vi "CustomerSpecific_SendReceive.vi"(6 "error source":string="Diagnostic Service.vi", 8 "error in (no error)":errorcluster, 9 "data in":u8[](array[numeric]), 10 "require response?":bool=TRUE, 11 "diag ref in":T1={"Diag CAN Handle"=0, "Transport Protocol"=enum."ISO TP - Normal Mode", "Receive Address Extension"=0, "Transmit Address Extension"=0, "Receive CAN Id"=0, "Transmit CAN Id"=0, "Log Frames ?"=FALSE, "My TP Address"=0, "Other TP Address"=0, "T1"=0, "T2"=0, "T3"=0, "T4"=0, "Tx SN"=0, "Block Size"=0, "Rx SN"=0, "VW TP Initialized?"=FALSE, "Tx block no"=0, "baud rate"=0, "Interface"="", "Channel Diag CAN Handle"=0, "UDP Connection ID"=refnum, "TCP Connection ID"=refnum, "Target IP Addr"=0, "Source Address"=0, "Target Address"=0, "Send Header NACK?"=FALSE, "DLL Handle"=0, "NAD"=0, "Time Stamp read first"=0.0, "Time Stamp read last"=0.0, "Time Stamp write first"=0.0, "Time Stamp write last"=0.0, "Time Stamp write"=0.0, "Time Stamp read"=0.0, " I/O Mode"=0, "FD Baudrate"=0, "TX_DL"=8, "RX_DL"=8, "DoIP Protocol Version"=1, " Selected I/O Mode"=0, "TesterPresent Counter"=0, "TesterPresent Limit"=0, "TesterPresent Tick[ms]"=10, "TesterPresent RequireResponse?"=FALSE, "TesterPresent Stored Ref?"=FALSE, "TesterPresent Message"=[], "TesterPresent Task Handle"=0, "TesterPresent Semaphore"=refnum, "Response Plausibility Check"=1, "Default Version?"=TRUE, "Diagostic Globals"={"Timeout FC (Bs)"=250, "Timeout CF (Cr)"=250, "Timeout Diag Command"=1000, "Receive Block Size (BS)"=0, "Wait Time CF (STmin)"=5, "Max Waits (N_WFTmax)"=10, "Waits to Send (N_WAIT)"=0, "Time between Waits (TW)"=25, "Fill CAN Frames?"=TRUE, "Fill Byte"=255, "Invalid Response as Error?"=FALSE, "Max RspPending Count"=5, "VWTP Command Timeout"=50, "Transport Protocol"=enum."Diagnostics on IP", "Diag CAN Handle"=0, "DLL Handle"=0, "Timeout RspPending"=1000}, "Session-based Properties?"=FALSE, "NI-XNET IP Stack Reference"=0, "NI-XNET IP Stack TCP Reference"=-1, "NI-XNET IP Stack UDP Reference"=-1, "NI-XNET IP Stack Local Interface"="", "Functional CAN Id"=0, "Diag CAN Queue"=refnum, "Frame Fillling Mode"=0, "DoIP Acknowledge Mode"=0, "Message Buffer"=[]} {"Diagostic Globals"."Fill Byte" format="%x"; "TesterPresent Message" format="%.0x"; "Selected I/O Mode" items=["CAN", "CAN FD", "CAN FD+BRS", "ECU Determined"]; "DoIP Protocol Version" items=["2010"=1, "2012"=2]; "RX_DL" items=["8"=8, "12"=12, "16"=16, "20"=20, "24"=24, "32"=32, "48"=48, "64"=64]; "TX_DL" items=["8"=8, "12"=12, "16"=16, "20"=20, "24"=24, "32"=32, "48"=48, "64"=64]; "I/O Mode" items=["CAN", "CAN FD", "CAN FD+BRS", "Not yet determined"]}) -> (0 "error out":errorcluster, 1 "data out":u8[](array[numeric]), 2 "error code":u8, 3 "diag ref out":T1={"Diag CAN Handle"=0, "Transport Protocol"=enum."ISO TP - Normal Mode", "Receive Address Extension"=0, "Transmit Address Extension"=0, "Receive CAN Id"=0, "Transmit CAN Id"=0, "Log Frames ?"=FALSE, "My TP Address"=0, "Other TP Address"=0, "T1"=0, "T2"=0, "T3"=0, "T4"=0, "Tx SN"=0, "Block Size"=0, "Rx SN"=0, "VW TP Initialized?"=FALSE, "Tx block no"=0, "baud rate"=0, "Interface"="", "Channel Diag CAN Handle"=0, "UDP Connection ID"=refnum, "TCP Connection ID"=refnum, "Target IP Addr"=0, "Source Address"=0, "Target Address"=0, "Send Header NACK?"=FALSE, "DLL Handle"=0, "NAD"=0, "Time Stamp read first"=0.0, "Time Stamp read last"=0.0, "Time Stamp write first"=0.0, "Time Stamp write last"=0.0, "Time Stamp write"=0.0, "Time Stamp read"=0.0, " I/O Mode"=0, "FD Baudrate"=0, "TX_DL"=8, "RX_DL"=8, "DoIP Protocol Version"=1, " Selected I/O Mode"=0, "TesterPresent Counter"=0, "TesterPresent Limit"=0, "TesterPresent Tick[ms]"=10, "TesterPresent RequireResponse?"=FALSE, "TesterPresent Stored Ref?"=FALSE, "TesterPresent Message"=[], "TesterPresent Task Handle"=0, "TesterPresent Semaphore"=refnum, "Response Plausibility Check"=1, "Default Version?"=TRUE, "Diagostic Globals"={"Timeout FC (Bs)"=250, "Timeout CF (Cr)"=250, "Timeout Diag Command"=1000, "Receive Block Size (BS)"=0, "Wait Time CF (STmin)"=5, "Max Waits (N_WFTmax)"=10, "Waits to Send (N_WAIT)"=0, "Time between Waits (TW)"=25, "Fill CAN Frames?"=TRUE, "Fill Byte"=255, "Invalid Response as Error?"=FALSE, "Max RspPending Count"=5, "VWTP Command Timeout"=50, "Transport Protocol"=enum."Diagnostics on IP", "Diag CAN Handle"=0, "DLL Handle"=0, "Timeout RspPending"=1000}, "Session-based Properties?"=FALSE, "NI-XNET IP Stack Reference"=0, "NI-XNET IP Stack TCP Reference"=-1, "NI-XNET IP Stack UDP Reference"=-1, "NI-XNET IP Stack Local Interface"="", "Functional CAN Id"=0, "Diag CAN Queue"=refnum, "Frame Fillling Mode"=0, "DoIP Acknowledge Mode"=0, "Message Buffer"=[]} {"Diagostic Globals"."Fill Byte" format="%x"; "TesterPresent Message" format="%.0x"; "Selected I/O Mode" items=["CAN", "CAN FD", "CAN FD+BRS", "ECU Determined"]; "DoIP Protocol Version" items=["2010"=1, "2012"=2]; "RX_DL" items=["8"=8, "12"=12, "16"=16, "20"=20, "24"=24, "32"=32, "48"=48, "64"=64]; "TX_DL" items=["8"=8, "12"=12, "16"=16, "20"=20, "24"=24, "32"=32, "48"=48, "64"=64]; "I/O Mode" items=["CAN", "CAN FD", "CAN FD+BRS", "Not yet determined"]})   [LabVIEW 2024, in "Diagnostics Addon Engine.lvlib"]
uses:
  Diagnostics Addon Engine.lvlib
  <vilib>/Automotive Diagnostic Command Set/Diagnostic Transport.llb/Diag Reference.ctl
  <vilib>/Automotive Diagnostic Command Set/Diagnostic Transport.llb/Transport Protocol Selector.ctl
  <vilib>/Automotive Diagnostic Command Set/Diagnostic Transport.llb/DoIP Protocol Version.ctl
  <vilib>/Automotive Diagnostic Command Set/Diagnostic Transport.llb/Diag Globals.ctl
  <vilib>/Automotive Diagnostic Command Set/Diagnostic Transport.llb/ISOTP Recv Frame.vi
  <vilib>/Automotive Diagnostic Command Set/Diagnostic Transport.llb/ISOTP Recv CFs.vi
  <vilib>/Automotive Diagnostic Command Set/Diagnostic Transport.llb/ISOTP7 Recv Frame.vi
  <vilib>/Automotive Diagnostic Command Set/Diagnostic Transport.llb/ISOTP7 Recv CFs.vi
  <vilib>/Automotive Diagnostic Command Set/Diagnostic Transport.llb/ISOTP Send FF.vi
  <vilib>/Automotive Diagnostic Command Set/Diagnostic Transport.llb/ISOTP Send CFs.vi
  <vilib>/Automotive Diagnostic Command Set/Diagnostic Transport.llb/ISOTP Send Single Frame.vi
  <vilib>/Automotive Diagnostic Command Set/Diagnostic Transport.llb/Long CAN Frame Forced.vi
  <vilib>/Automotive Diagnostic Command Set/Diagnostic Transport.llb/ISOTP7 Send FF.vi
  <vilib>/Automotive Diagnostic Command Set/Diagnostic Transport.llb/ISOTP7 Send CFs.vi
  <vilib>/Automotive Diagnostic Command Set/Diagnostic Transport.llb/ISOTP7 Send Single Frame.vi
  <vilib>/Automotive Diagnostic Command Set/Diagnostic Transport.llb/ISOTP Check Redo.vi
  <vilib>/Automotive Diagnostic Command Set/Diagnostic Transport.llb/ISOTP Recv Block.vi
  <vilib>/Automotive Diagnostic Command Set/Diagnostic Transport.llb/ISOTP7 Recv Block.vi
  <vilib>/Automotive Diagnostic Command Set/Diagnostic Transport.llb/ISOTP Send Frame.vi
  <vilib>/Automotive Diagnostic Command Set/Diagnostic Transport.llb/ISOTP Recv FC.vi
  <vilib>/Automotive Diagnostic Command Set/Diagnostic Transport.llb/ISOTP Send CF.vi
  <vilib>/Automotive Diagnostic Command Set/Diagnostic Transport.llb/Diag Fill Frame.vi
  <vilib>/Automotive Diagnostic Command Set/Diagnostic Transport.llb/ISOTP Calc Send Params.vi
  <vilib>/Automotive Diagnostic Command Set/Diagnostic Transport.llb/Diag Get Globals.vi
  <vilib>/Automotive Diagnostic Command Set/Diagnostic Transport.llb/ISOTP7 Send Frame.vi
  <vilib>/Automotive Diagnostic Command Set/Diagnostic Transport.llb/ISOTP7 Recv FC.vi
  <vilib>/Automotive Diagnostic Command Set/Diagnostic Transport.llb/ISOTP7 Send CF.vi
  <vilib>/Automotive Diagnostic Command Set/Diagnostic Transport.llb/ISOTP Send FC.vi
  <vilib>/Automotive Diagnostic Command Set/Diagnostic Transport.llb/ISOTP Add CF.vi
  <vilib>/Automotive Diagnostic Command Set/Diagnostic Transport.llb/ISOTP7 Send FC.vi
  <vilib>/Automotive Diagnostic Command Set/Diagnostic Transport.llb/ISOTP7 Add CF.vi
  <vilib>/Automotive Diagnostic Command Set/Diagnostic Transport.llb/Diag Globals.vi
  <vilib>/Automotive Diagnostic Command Set/Diagnostic Transport.llb/CAN Send Frame Check Queue.vi
  <vilib>/Automotive Diagnostic Command Set/Diagnostic Transport.llb/Diag CAN get timestamp.vi
  <vilib>/Automotive Diagnostic Command Set/Diagnostic Transport.llb/Diag CAN read.vi
  <vilib>/Automotive Diagnostic Command Set/Diagnostic Transport.llb/ISOTP Calc Actual IO Mode.vi
  <vilib>/Automotive Diagnostic Command Set/Diagnostic Transport.llb/ISOTP Get FC Data.vi
  <vilib>/addons/Automotive Diagnostic Command Set/NI_Automotive Diagnostic Command Set.lvlib
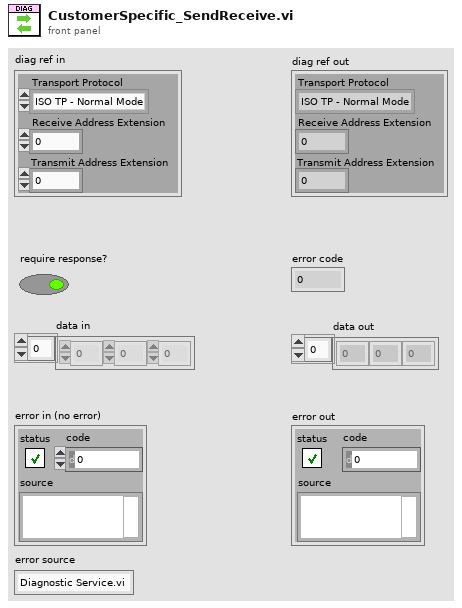
[diagram p1: front panel]
types:
  T1 = typedef "NI_Automotive Diagnostic Command Set.lvlib/Diag Reference.ctl" = cluster{"Diag CAN Handle":u32, "Transport Protocol":T2, "Receive Address Extension":u8, "Transmit Address Extension":u8, "Receive CAN Id":u32, "Transmit CAN Id":u32, "Log Frames ?":bool, "My TP Address":u8, "Other TP Address":u8, "T1":u16, "T2":u16, "T3":u16, "T4":u16, "Tx SN":u8, "Block Size":u8, "Rx SN":u8, "VW TP Initialized?":bool, "Tx block no":u8, "baud rate":u64, "Interface":string, "Channel Diag CAN Handle":u32, "UDP Connection ID":refnum<k16>, "TCP Connection ID":refnum<k5>, "Target IP Addr":u32, "Source Address":u16, "Target Address":u16, "Send Header NACK?":bool, "DLL Handle":u32, "NAD":u8, "Time Stamp read first":dbl, "Time Stamp read last":dbl, "Time Stamp write first":dbl, "Time Stamp write last":dbl, "Time Stamp write":dbl, "Time Stamp read":dbl, " I/O Mode":u32, "FD Baudrate":u64, "TX_DL":u16, "RX_DL":u16, "DoIP Protocol Version":T3, " Selected I/O Mode":u32, "TesterPresent Counter":u32, "TesterPresent Limit":u32, "TesterPresent Tick[ms]":i32, "TesterPresent RequireResponse?":bool, "TesterPresent Stored Ref?":bool, "TesterPresent Message":u8[], "TesterPresent Task Handle":i32, "TesterPresent Semaphore":T4, "Response Plausibility Check":u32, "Default Version?":bool, "Diagostic Globals":T5, "Session-based Properties?":bool, "NI-XNET IP Stack Reference":i64, "NI-XNET IP Stack TCP Reference":i64, "NI-XNET IP Stack UDP Reference":i64, "NI-XNET IP Stack Local Interface":string, "Functional CAN Id":u32, "Diag CAN Queue":refnum<queue>, "Frame Fillling Mode":u32, "DoIP Acknowledge Mode":u32, "Message Buffer":u8[]}
  T2 = typedef "NI_Automotive Diagnostic Command Set.lvlib/Transport Protocol Selector.ctl" = enum16{"ISO TP - Normal Mode", "ISO TP - Mixed Mode", "VW TP 2.0", "Diagnostics on IP", "ISO TP LIN"}
  T3 = typedef "NI_Automotive Diagnostic Command Set.lvlib/DoIP Protocol Version.ctl" = u8
  T4 = typedef "Semaphore RefNum" = refnum<k1>
  T5 = typedef "NI_Automotive Diagnostic Command Set.lvlib/Diag Globals.ctl" = cluster{"Timeout FC (Bs)":u32, "Timeout CF (Cr)":u32, "Timeout Diag Command":u32, "Receive Block Size (BS)":u8, "Wait Time CF (STmin)":u8, "Max Waits (N_WFTmax)":u8, "Waits to Send (N_WAIT)":i32, "Time between Waits (TW)":u32, "Fill CAN Frames?":bool, "Fill Byte":u32, "Invalid Response as Error?":bool, "Max RspPending Count":u32, "VWTP Command Timeout":u32, "Transport Protocol":T2, "Diag CAN Handle":u32, "DLL Handle":u32, "Timeout RspPending":u32}
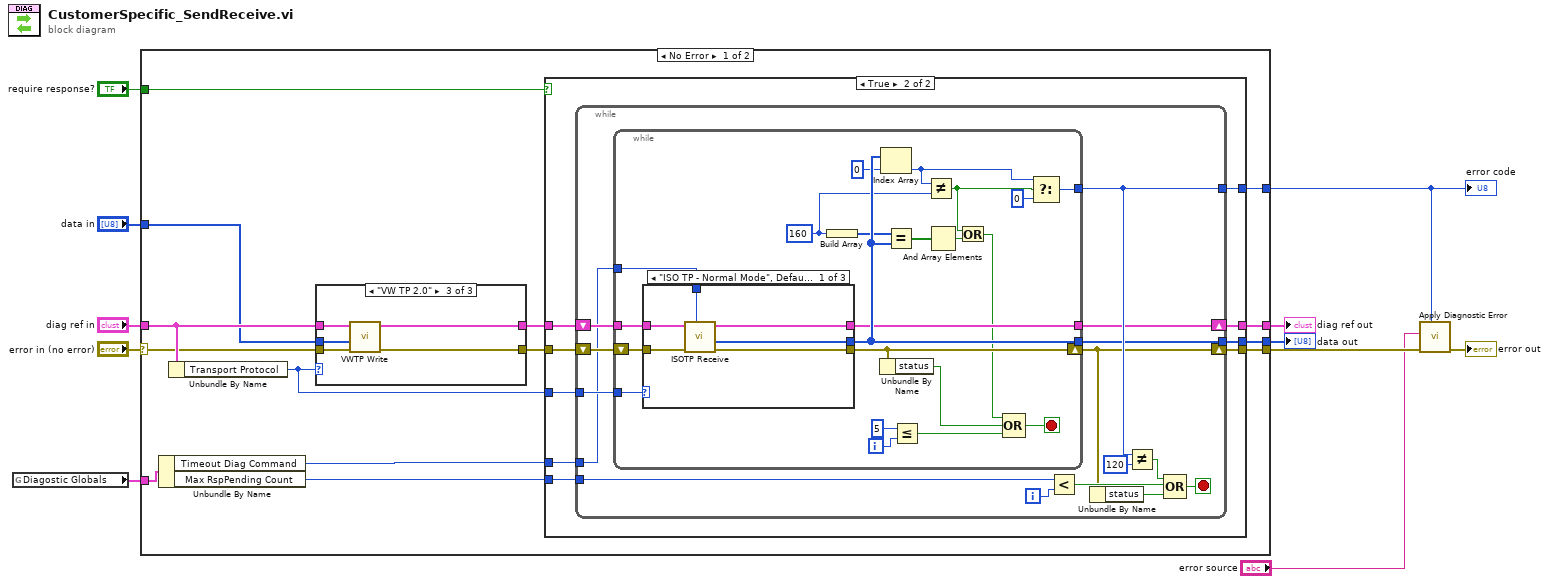
[diagram p0: block diagram]
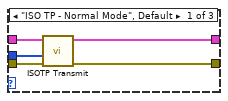
[diagram p2: hidden frame]
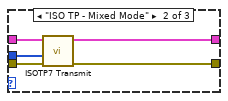
[diagram p3: hidden frame]
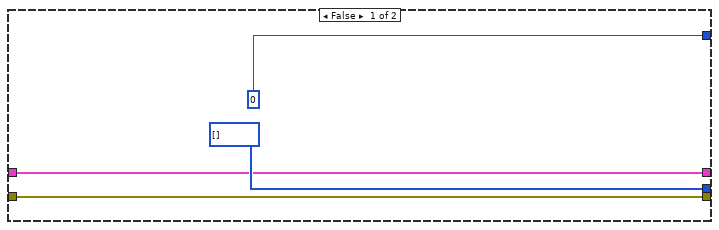
[diagram p4: hidden frame]
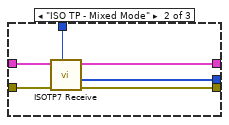
[diagram p5: hidden frame]
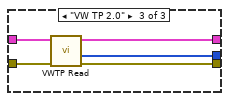
[diagram p6: hidden frame]
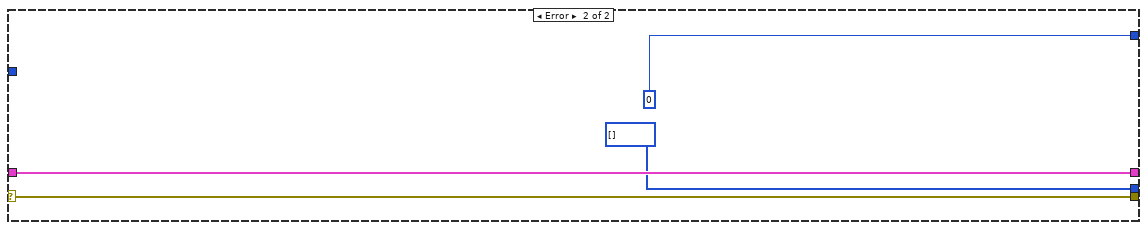
[diagram p7: hidden frame]
diagram:
  n1 = global read "Diag Globals.vi" "Diagostic Globals"() -> (w2:T5)
  n2 = case shown="No Error" "error in (no error)" {
    selector: "error in (no error)" -> [w19 w110]
    tunnel: "data in" -> [w18 _]
    tunnel: [w25 u8[] [] ("data out")] -> w5
    tunnel: [w24 w111] -> w1
    tunnel: [w23 w110] -> w11
    tunnel: "diag ref in" -> [w20 w111]
    tunnel: [w22 u8 0 ("error code")] -> w8
    tunnel: "require response?" -> [w21 _]
    tunnel: w2 -> [w15 _]
    frame No Error {
      n3 = Unbundle By Name(w15) -> ("Timeout Diag Command"=w12:u32, "Max RspPending Count"=w14:u32)
      n4 = Unbundle By Name(w20) -> ("Transport Protocol"=w13:T2)
      n5 = case shown="\"VW TP 2.0\"" w13 {
        tunnel: w19 -> [w30 w35 w39]
        tunnel: w18 -> [w29 w34 w36]
        tunnel: [w27 w32 w38] -> w16
        tunnel: w20 -> [w28 w33 w40]
        tunnel: [w26 w31 w37] -> w17
        frame "ISO TP - Normal Mode", Default {
          n6 = call <vilib>:"ISOTP Transmit.vi"("error in (no error)"=w30, "data"=w29, "diag ref in"=w28) -> ("error out"=w26:errorcluster, "diag ref out"=w27:T1)  [unwired: 7 in]
        }
        frame "ISO TP - Mixed Mode" {
          n7 = call <vilib>:"ISOTP7 Transmit.vi"("error in (no error)"=w35, "data"=w34, "diag ref in"=w33) -> ("error out"=w31:errorcluster, "diag ref out"=w32:T1)  [unwired: 7 in]
        }
        frame "VW TP 2.0" {
          n8 = call <vilib>:"VWTP Write.vi"("error in"=w39, "data in"=w36, "diag ref in"=w40) -> ("error out"=w37:errorcluster, "diag ref out"=w38:T1)  [unwired: 7 in]
        }
      }
      n9 = case shown="True" w21 {
        tunnel: [u8[] [] ("data out") w53] -> w25
        tunnel: [w43 w52] -> w24
        tunnel: [w42 w51] -> w23
        tunnel: w16 -> [w43 w50]
        tunnel: w17 -> [w42 w49]
        tunnel: [u8 0 ("error code") w48] -> w22
        tunnel: w14 -> [_ w47]
        tunnel: w13 -> [_ w46]
        tunnel: w12 -> [_ w45]
        frame False {
        }
        frame True {
          n10 = while {
            tunnel: [w58] -> w53
            shift-right: [w57] -> w51
            shift-left: w49 -> [w61]
            tunnel: [w59] -> w48
            shift-right: [w56] -> w52
            shift-left: w50 -> [w60]
            tunnel: w47 -> [w62]
            tunnel: w46 -> [w55]
            tunnel: w45 -> [w54]
            i -> [w64]
            stop <- w67 stop-if-true
            n11 = while {
              tunnel: [w84] -> w58
              tunnel: [w81] -> w56
              tunnel: w60 -> [w85]
              tunnel: [w83] -> w59
              shift-right: [w82] -> w57
              shift-left: w61 -> [w86]
              tunnel: w55 -> [w78]
              tunnel: w54 -> [w77]
              i -> [w87]
              stop <- w90 stop-if-true
              w75 = u8 160 ("element")
              n12 = case shown="\"ISO TP - Normal Mode\", Default" w78 {
                tunnel: w86 -> [w91 w97 w106]
                tunnel: [w96 w102 w103] -> w84
                tunnel: [w95 w101 w104] -> w81
                tunnel: w85 -> [w92 w98 w107]
                tunnel: [w94 w100 w105] -> w82
                tunnel: w77 -> [w93 w99 _]
                frame "ISO TP - Normal Mode", Default {
                  n13 = call <vilib>:"ISOTP Receive.vi"("timeout [ms]"=w93, "error in (no error)"=w91, "diag ref in"=w92) -> ("error out"=w94:errorcluster, "data"=w96:u8[], "diag ref out"=w95:T1)  [unwired: 6 in]
                }
                frame "ISO TP - Mixed Mode" {
                  n14 = call <vilib>:"ISOTP7 Receive.vi"("timeout [ms]"=w99, "error in (no error)"=w97, "diag ref in"=w98) -> ("error out"=w100:errorcluster, "data"=w102:u8[], "diag ref out"=w101:T1)  [unwired: 6 in]
                }
                frame "VW TP 2.0" {
                  n15 = call <vilib>:"VWTP Read.vi"("error in"=w106, "diag ref in"=w107) -> ("error out"=w105:errorcluster, "data out"=w103:u8[], "diag ref out"=w104:T1)  [unwired: 7 in]
                }
              }
              n16 = Build Array(w75) -> (w76:u8[])
              n17 = Unbundle By Name(w82) -> ("status"=w79:bool)
              n18 = Index Array(array=w84, index=0) -> (element=w70:u8)
              n19 = Equal?(x=w76, y=w84) -> (x = y?=w73:bool[])
              n20 = Less Or Equal?(x=5, y=w87) -> (x <= y?=w88:bool)
              n21 = Not Equal?(x=w70, y=w75) -> (x != y?=w71:bool)
              n22 = And Array Elements(Boolean array=w73) -> (logical AND=w72:bool)
              n23 = Or(x=w71, y=w72) -> (x .or. y?=w80:bool)
              n24 = Compound Arithmetic op=OR(w80, w79, w88) -> (w90:bool)
              n25 = Select(t=w70, s=w71, f=u8 0) -> (s? t:f=w83:u8)
            }
            n26 = Less?(x=w62, y=w64) -> (x < y?=w63:bool)
            n27 = Unbundle By Name(w57) -> ("status"=w66:bool)
            n28 = Not Equal?(x=w59, y=u8 120) -> (x != y?=w65:bool)
            n29 = Compound Arithmetic op=OR(w65, w63, w66) -> (w67:bool)
          }
        }
      }
    }
    frame Error {
    }
  }
  "data out" <- w5
  "error code" <- w8
  "diag ref out" <- w1
  n30 = call <vilib>:"Apply Diagnostic Error.vi"("error code"=w8, "error in (no error)"=w11, "error source"="error source") -> ("error out"=→"error out":errorcluster)  [unwired: 8 in]
